vi "Untitled 2 (SubVI).vi"(8 "Numeric 5":dbl, 11 "Numeric 6":dbl) -> (2 "Numeric":dbl)   [LabVIEW 2022 SP3]
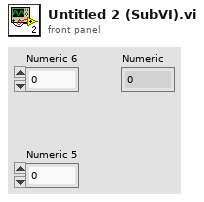
[diagram p1: front panel]
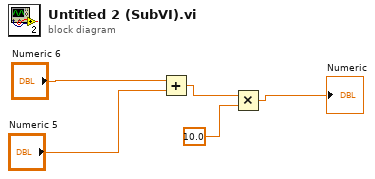
[diagram p0: block diagram]
diagram:
  n1 = Add(x="Numeric 6", y="Numeric 5") -> (x+y=w2:dbl)
  n2 = Multiply(x=w2, y=10.0) -> (x*y=→"Numeric":dbl)
